vi "ReciveBuffer.vi"(1 "销毁?":bool) -> (0 "VCI_USB_CAN_T_BUF_R":refnum<queue>)   [LabVIEW 2011]
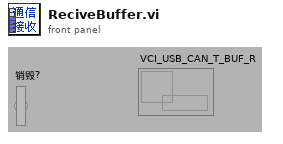
[diagram p1: front panel]
types:
  T1 = cluster{"time":timestamp, "channel":u16, "tr":enum16{"接收", "发送"}, "id":u32, "Type":enum16{"数据帧", "远程帧"}, "Format":enum16{"标准帧", "扩展帧"}, "len":u8, "data":u8[]}
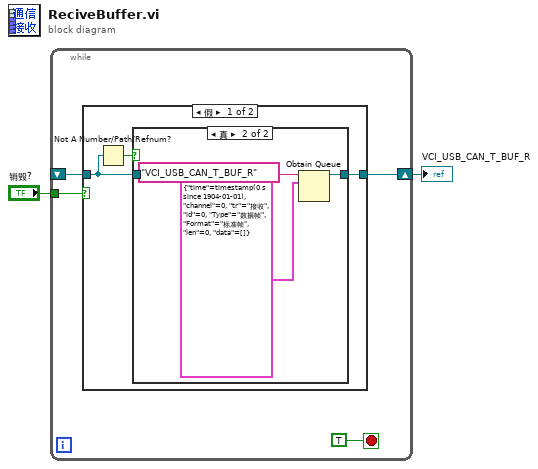
[diagram p0: block diagram]
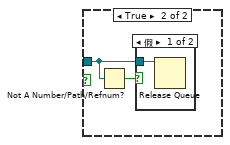
[diagram p3: hidden frame]
diagram:
  n1 = while {
    shift-right: [w4] -> w1
    shift-left: _ -> [w5]
    tunnel: "销毁?" -> [w3]
    stop <- TRUE stop-if-true
    n2 = case shown="假" w3 {
      tunnel: w5 -> [w8 w14]
      tunnel: [w7 _] -> w4
      frame False {
        n3 = Not A Number/Path/Refnum?(number/path/refnum=w8) -> (NaN/Path/Refnum?=w9:bool)
        n4 = case shown="真" w9 {
          tunnel: w8 -> [w10 _]
          tunnel: [w10 w12] -> w7
          frame False {
          }
          frame True {
            n5 = Obtain Queue(name (unnamed)="VCI_USB_CAN_T_BUF_R" ("名称（未命名）"), element data type=T1 {"time"=timestamp(0 s since 1904-01-01), "channel"=0, "tr"=enum."接收", "id"=0, "Type"=enum."数据帧", "Format"=enum."标准帧", "len"=0, "data"=[]} ("TR_Unit")) -> (queue out=w12:refnum<queue>)  [unwired: 3 in, 2 out]
          }
        }
      }
      frame True {
        n6 = Not A Number/Path/Refnum?(number/path/refnum=w14) -> (NaN/Path/Refnum?=w15:bool)
        n7 = case shown="假" w15 {
          tunnel: w14 -> [w16 _]
          frame False {
            n8 = Release Queue(queue=w16) -> ()  [unwired: 2 in, 3 out]
          }
          frame True {
          }
        }
      }
    }
  }
  "VCI_USB_CAN_T_BUF_R" <- w1
